vi "Load Experiment File.vi"(8 "error in (no error)":errorcluster, 11 "Experiment File Path":path) -> (0 "error out":errorcluster, 1 "Experiment Name":string, 2 "Experiment File out":T1, 3 "Experiment File Path out (duplicate)":path)   [LabVIEW 2020, in "Experiment File.lvlib"]
doc: "Load the given project file or open a file dialog if no path is given. To aid in backwards compatability as new features are added, if a setting is not found in the file, the error is ignored and the undiscovered setting is set to a default value."
uses:
  Experiment File.lvlib
  Experiment File Cluster.ctl
  Plugin Servers/Controller/Minimal Controller Cluster.ctl
  Plugin Servers/Parameter to Hardware Map/Minimal Map.ctl
  Plugin Servers/Parameter to Hardware Map/Minimal Pair Cluster.ctl
  Plugin Servers/Controller/Generic Plugin.lvclass
  Plugin Servers/Parameter to Hardware Map/Parameter to Hardware Map.lvclass
panel:
  out "text":string
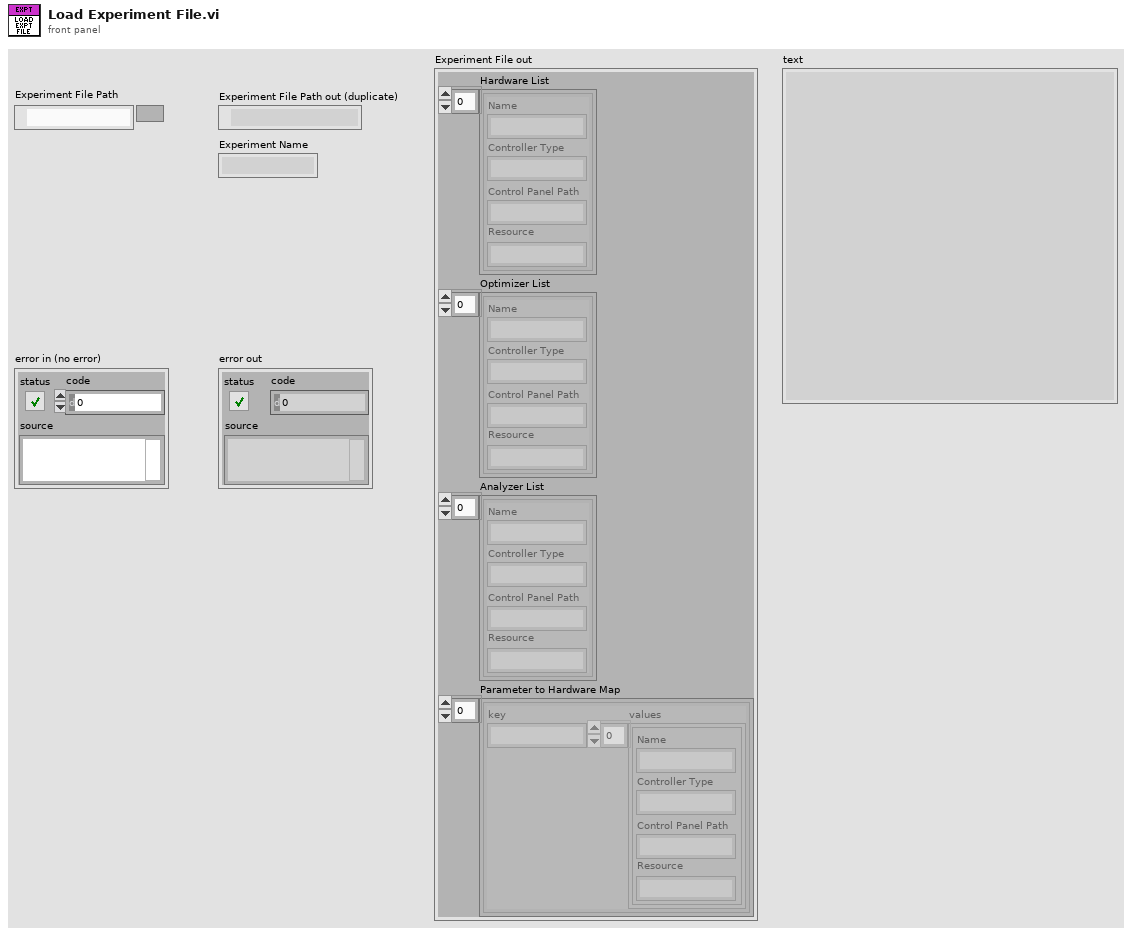
[diagram p1: front panel]
types:
  T1 = typedef "Experiment File.lvlib/Experiment File Cluster.ctl" = cluster{"Hardware List":T2[], "Optimizer List":T2[], "Analyzer List":T2[], "Parameter to Hardware Map":T3}
  T2 = typedef "Generic Plugin.lvclass/Minimal Controller Cluster.ctl" = cluster{"Name":string, "Controller Type":string, "Control Panel Path":string, "Resource":string}
  T3 = typedef "Parameter to Hardware Map.lvclass/Minimal Map.ctl" = T4[]
  T4 = typedef "Parameter to Hardware Map.lvclass/Minimal Pair Cluster.ctl" = cluster{"key":string, "values":T2[]}
  T5 = enum16{"open", "replace", "create", "open or create", "replace or create", "replace or create with confirmation"}
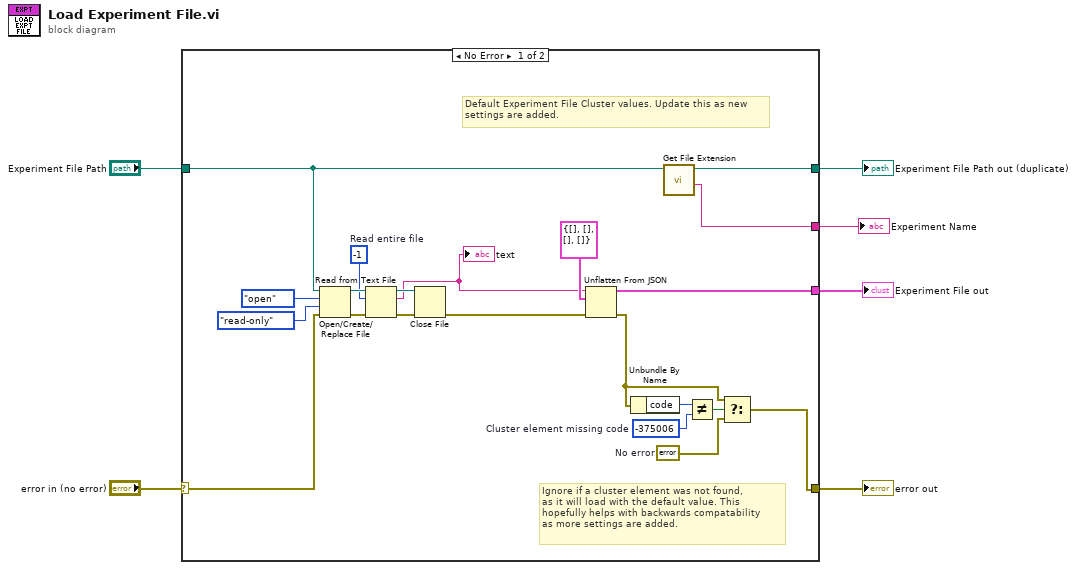
[diagram p0: block diagram]
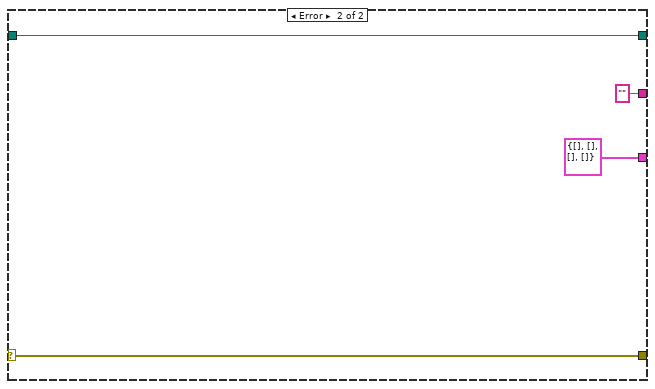
[diagram p2: hidden frame]
diagram:
  n1 = case shown="No Error" "error in (no error)" {
    selector: "error in (no error)" -> [w20 w31]
    tunnel: [w15 w31] -> w5
    tunnel: "Experiment File Path" -> [w9 w29]
    tunnel: [w26 T1 {"Hardware List"=[], "Optimizer List"=[], "Analyzer List"=[], "Parameter to Hardware Map"=[]} ("File")] -> w3
    tunnel: [w8 w29] -> w2
    tunnel: [w7 "" ("filename without extension")] -> w1
    frame No Error {
      w10 = errorcluster {"status"=FALSE, "code"=0, "source"=""}  # No error
      w13 = -375006  # Cluster element missing code
      w16 = -1  # Read entire file
      # "Default Experiment File Cluster values. Update this as new\nsettings are added."
      # "Ignore if a cluster element was not found,\nas it will load with the default value. This\nhopefully helps with backwards compatability\nas more settings are added."
      n2 = Open/Create/Replace File(file path (use dialog)=w9, error in=w20, operation (0:open)=T5."open", access (0:read/write)=enum16{"read/write", "read-only", "write-only"}."read-only") -> (refnum out=w22:refnum<file>, error out=w23:errorcluster)  [unwired: 2 in, 1 out]
      n3 = Read from Text File(file (use dialog)=w22, count=w16, error in=w23) -> (refnum out=w24:refnum<file>, text=w19:string, error out=w25:errorcluster)  [unwired: 1 in, 1 out]
      "text" <- w19
      n4 = Close File(refnum=w24, error in=w25) -> (error out=w21:errorcluster)  [unwired: 1 out]
      n5 = Unflatten From JSON(JSON string=w19, type and defaults=T1 {"Hardware List"=[], "Optimizer List"=[], "Analyzer List"=[], "Parameter to Hardware Map"=[]} ("File"), error in (no error)=w21) -> (value=w26:T1, error out=w11:errorcluster)  [unwired: 4 in]
      n6 = Unbundle By Name(w11) -> ("code"=w14:i32)
      n7 = call <vilib>:"Get File Extension.vi"("file"=w9) -> ("filename without extension"=w7:string, "dup file"=w8:path)  [unwired: 6 in, 3 out]
      n8 = Not Equal?(x=w14, y=w13) -> (x != y?=w12:bool)
      n9 = Select(t=w11, s=w12, f=w10) -> (s? t:f=w15:errorcluster)
    }
    frame Error {
    }
  }
  "error out" <- w5
  "Experiment File out" <- w3
  "Experiment File Path out (duplicate)" <- w2
  "Experiment Name" <- w1
